vi "unregisterRunEvents.vi"(8 "error in (no error)":errorcluster, 11 "ExperimentControlEvents in":refnum<class "ExperimentControlEvents.lvclass">) -> (0 "error out":errorcluster, 3 "ExperimentControlEvents out":refnum<class "ExperimentControlEvents.lvclass">)   [LabVIEW 2011, in "Views.lvlib" / "ExperimentControl.lvlib" / "ExperimentControlEvents.lvclass"]
uses:
  ExperimentControlEvents.lvclass
  Events/Event.lvclass
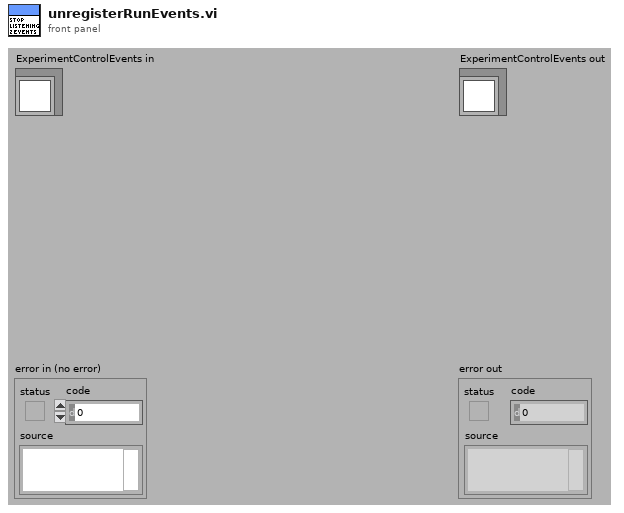
[diagram p1: front panel]
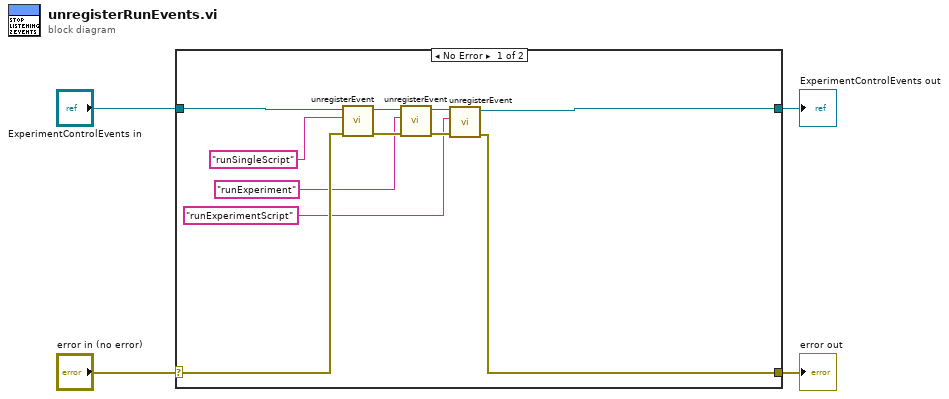
[diagram p0: block diagram]
diagram:
  n1 = case shown="No Error" "error in (no error)" {
    selector: "error in (no error)" -> [w14 w17]
    tunnel: [w10 w17] -> w3
    tunnel: [w11 w16] -> w1
    tunnel: "ExperimentControlEvents in" -> [w15 w16]
    frame No Error {
      n2 = call "unregisterEvent.vi"("error in (no error)"=w14, "name"="runSingleScript", "Event in"=w15) -> ("error out"=w8:errorcluster, "Event out"=w13:refnum<class "ExperimentControlEvents.lvclass">)  [unwired: 7 in]
      n3 = call "unregisterEvent.vi"("error in (no error)"=w8, "name"="runExperiment", "Event in"=w13) -> ("error out"=w9:errorcluster, "Event out"=w12:refnum<class "ExperimentControlEvents.lvclass">)  [unwired: 7 in]
      n4 = call "unregisterEvent.vi"("error in (no error)"=w9, "name"="runExperimentScript", "Event in"=w12) -> ("error out"=w10:errorcluster, "Event out"=w11:refnum<class "ExperimentControlEvents.lvclass">)  [unwired: 7 in]
    }
    frame Error {
    }
  }
  "error out" <- w3
  "ExperimentControlEvents out" <- w1
